vi "Cont Acq AI Samples-Int Clk-Init.vi"(8 "error in":errorcluster, 10 "Rate":dbl=1000.0 format="%0.2f", 11 "physical channels":tag) -> (0 "error out":errorcluster, 3 "AI task out":refnum<k21>)   [LabVIEW 2009]
doc: "I. Description:\nThis example demonstrates how to make continuous, hardware-timed temperature measurement using a thermocouple.\n\nII. Instructions for Running:\n1. Specify the Physical Channel where you have connected the thermocouple.\n2. Enter the Minimum and Maximum temperature values in degrees C you expect to measure. A smaller range will allow a more accurate measurement.\n3. Enter the scan rate at which you want to run the acquisition.\n4. Specify the type of thermocouple you are using.\n5. Thermocouple measurements require cold-junction compensation (CJC) to correctly scale them. Specify the source of your cold-junction compensation.\n6. If your CJC source is \"Internal\", skip the rest of the steps.\n7. If your CJC source is \"Constant Value\", specify the value (usually room temperature) in degrees C.\n8. If your CJC source is \"Channel\", specify the CJC Channel name. \n9. Specify the appropriate Auto Zero Mode. See your device's hardware manual to find out if your device supports this attribute.\n\nIII. Block Diagram Steps:\n1. Create a Thermocouple (TC) temperature measurement channel.\n2. Get all the channels in the task.\n3. Convert channel(s) array to a comma-delimited channel string.\n4. This attribute is set to compensate for input offset errors. May not be supported by all devices*.\n5. Call the Timing VI to specify the hardware timing parameters. Use device's internal clock, continuous mode acquisition and the sample rate specified by the user.\n6. Call the Start VI to program and start the acquisition.\n7. Read N samples and plot it. By default, the Read VI reads all available samples, but you can specify how many samples to read at a time and the timeout value. Continue reading data until the stop button is pressed or an error occurs. \n8. Call the Clear Task VI to clear the Task.\n9. Use the popup dialog box to display an error if any.\n\n* If your device does not support Auto Zero Mode bypass Step 2, 3, and 4.\n\nIV. I/O Connections Overview:\nConnect your thermocouple to the terminals corresponding to the Physical Channel I/O Control value."
uses:
  <vilib>/DAQmx/configure/timing.llb/DAQmx Timing (Sample Clock).vi
  <vilib>/DAQmx/create/channels.llb/DAQmx Create Channel (AI-Voltage-Basic).vi
  <vilib>/Utility/error.llb/DialogType.ctl
  <vilib>/DAQmx/read.llb/DAQmx Read (Analog 1D Wfm NChan NSamp).vi
  Program Files/National Instruments/LabVIEW 2009/resource/objmgr/daqmx.rc
panel:
  out "Measurement":waveform(dbl)[](graph)
  in  "stop":bool
  in  "Samples to Read":i32=-1
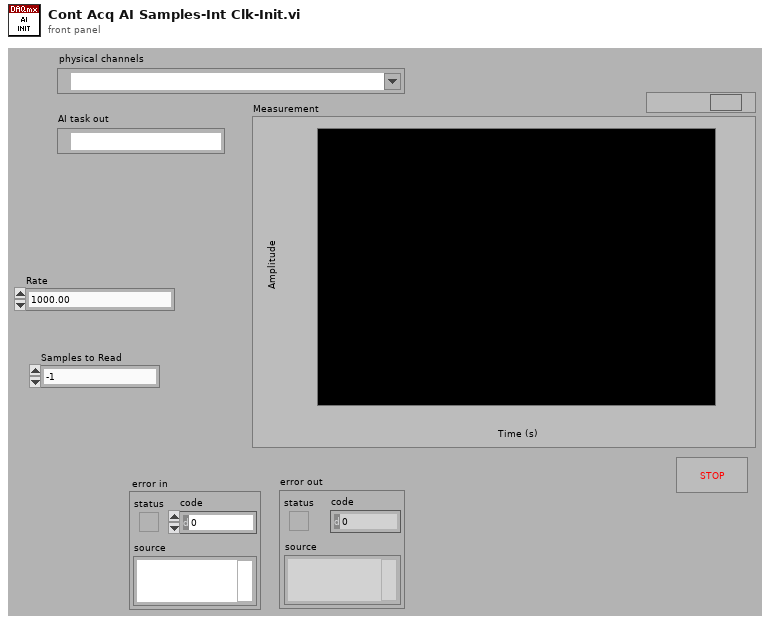
[diagram p1: front panel]
types:
  T1 = typedef "DialogType.ctl" = u16
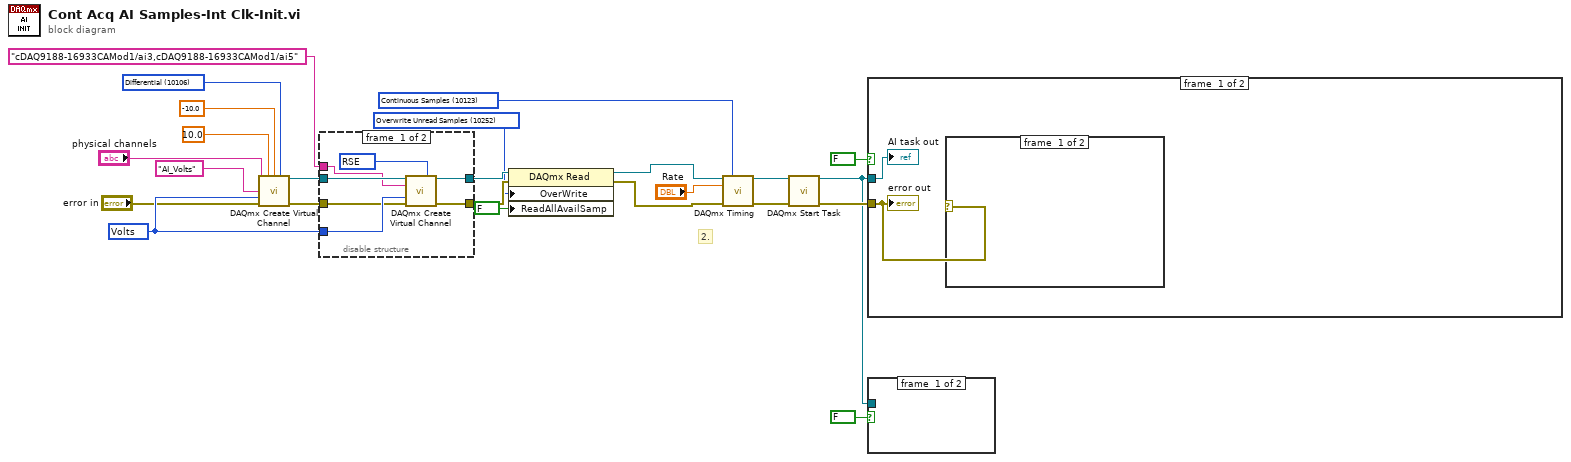
[diagram p0: block diagram]
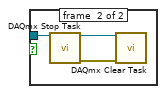
[diagram p2: hidden frame]
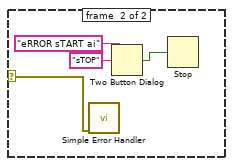
[diagram p4: hidden frame]
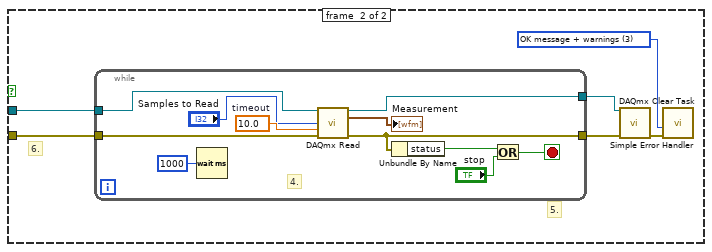
[diagram p5: hidden frame]
diagram:
  w2 = 10252 items=["Overwrite Unread Samples"=10252, "Do Not Overwrite Unread Samples"=10159] ("OverWrite")
  w9 = 10106 items=["default"=-1, "RSE"=10083, "NRSE"=10078, "Differential"=10106, "Pseudodifferential"=12529] ("input terminal configuration")
  w16 = 10348 items=["Volts"=10348, "From Custom Scale"=10065] ("units")
  w22 = 10123 items=["Finite Samples"=10178, "Continuous Samples"=10123] ("sample mode")
  # "2."
  n1 = call-poly <vilib>:"DAQmx Create Virtual Channel.vi"("maximum value"=10.0, "minimum value"=-10.0, "input terminal configuration"=w9, "physical channels"="physical channels", "name to assign"="AI_Volts", "units"=w16, "error in"="error in") -> ("task out"=w18:refnum<k21>, "error out"=w14:errorcluster)  [unwired: 7 in]
  n2 = disable-structure shown="Enabled" {
    disable-tunnel: w18 -> [w31 w32]
    disable-tunnel: "cDAQ9188-16933CAMod1/ai3,cDAQ9188-16933CAMod1/ai5" -> [w29 _]
    disable-tunnel: w16 -> [w28 _]
    disable-tunnel: w14 -> [w27 w33]
    disable-tunnel: [w26 w32] -> w6
    disable-tunnel: [w25 w33] -> w3
    frame #0 {
      w30 = 10083 items=["default"=-1, "RSE"=10083, "NRSE"=10078, "Differential"=10106, "Pseudodifferential"=12529] ("input terminal configuration")
      n3 = call-poly <vilib>:"DAQmx Create Virtual Channel.vi"("task in"=w31, "input terminal configuration"=w30, "physical channels"=w29, "units"=w28, "error in"=w27) -> ("task out"=w26:refnum<k21>, "error out"=w25:errorcluster)  [unwired: 9 in]
    }
    frame #1 {
    }
  }
  n4 = property class="DAQmx Read"(reference=w6, error in=w3, "OverWrite"=w2, "ReadAllAvailSamp"=FALSE) -> (reference out=w5:refnum<k21>, error out=w4:errorcluster)
  n5 = call-poly <vilib>:"DAQmx Timing.vi"("task/channels in"=w5, "sample mode"=w22, "rate"="Rate", "error in"=w4) -> ("task out"=w23:refnum<k21>, "error out"=w24:errorcluster)  [unwired: 10 in]
  n6 = call <vilib>:"DAQmx Start Task.vi"("task/channels in"=w23, "error in"=w24) -> ("task out"=w12:refnum<k21>, "error out"=w21:errorcluster)  [unwired: 12 in]
  n7 = case shown="False" FALSE {
    tunnel: w12 -> [w35 w42]
    tunnel: w21 -> [w34 w40]
    frame #0 {
      n8 = case shown="Error" w34 {
        selector: w34 -> [_ w39]
        frame #0 {
        }
        frame #1 {
          n9 = call <vilib>:"Simple Error Handler.vi"("error in (no error)"=w39) -> ()  [unwired: 4 in, 5 out]
          n10 = Two Button Dialog(message="eRROR sTART ai", 2:"sTOP" ("T button name (\"OK\")")) -> (T button?=w38:bool)  [unwired: 1 in]
          n11 = Stop(stop? (T)=w38) -> ()
        }
      }
      "error out" <- w34
      "AI task out" <- w35
    }
    frame #1 {
      w45 = T1 3 items=["no dialog", "OK message", "continue or stop message", "OK message + warnings", "continue/stop + warnings"] ("type of dialog (OK msg:1)")
      # "6."
      # "5."
      n12 = while {
        tunnel: w40 -> [w56]
        tunnel: w42 -> [w55]
        tunnel: [w54] -> w43
        tunnel: [w52] -> w44
        stop <- w50 stop-if-true
        w48 = 10.0  # timeout
        # "4."
        n13 = Wait (ms)(milliseconds to wait=u32 1000) -> ()  [unwired: 1 out]
        n14 = call-poly <vilib>:"DAQmx Read.vi"("task/channels in"=w55, "number of samples per channel"="Samples to Read", "timeout"=w48, "error in"=w56) -> ("task out"=w54:refnum<k21>, "data"=→"Measurement":waveform(dbl)[], "error out"=w52:errorcluster)  [unwired: 9 in]
        n15 = Unbundle By Name(w52) -> ("status"=w51:bool)
        n16 = Or(x=w51, y="stop") -> (x .or. y?=w50:bool)
      }
      n17 = call <vilib>:"DAQmx Clear Task.vi"("task in"=w43, "error in"=w44) -> ("error out"=w41:errorcluster)  [unwired: 13 in]
      n18 = call <vilib>:"Simple Error Handler.vi"("type of dialog (OK msg:1)"=w45, "error in (no error)"=w41) -> ()  [unwired: 3 in, 5 out]
    }
  }
  n19 = case shown="True" FALSE {
    tunnel: w12 -> [_ w57]
    frame #0 {
    }
    frame #1 {
      n20 = call <vilib>:"DAQmx Stop Task.vi"("task/channels in"=w57) -> ("task out"=w59:refnum<k21>, "error out"=w58:errorcluster)  [unwired: 13 in]
      n21 = call <vilib>:"DAQmx Clear Task.vi"("task in"=w59, "error in"=w58) -> ()  [unwired: 13 in, 1 out]
    }
  }
